vi "TagDB-Obtain.vi"(4 "error in (no error)":errorcluster, 6 "name (unnamed)":string) -> (0 "error out":errorcluster, 1 "created new?":bool, 3 "TagDB":refnum<k1>)   [LabVIEW 2017, in "TagDB.lvlib"]
uses:
  TagDB.lvlib
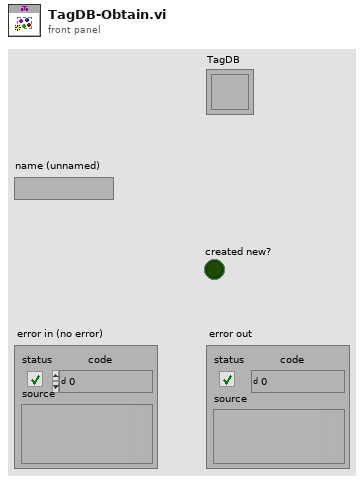
[diagram p1: front panel]
types:
  T1 = enum16{"create", "destroy", "cleanUp", "list", "get info", "force destroy"}
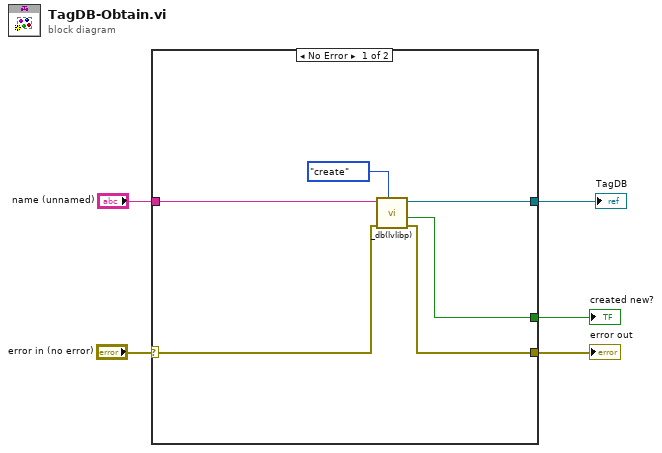
[diagram p0: block diagram]
diagram:
  n1 = case shown="No Error" "error in (no error)" {
    selector: "error in (no error)" -> [w6 w12]
    tunnel: [w10 w12] -> w2
    tunnel: [w9 _] -> w1
    tunnel: [w11 _] -> w3
    tunnel: "name (unnamed)" -> [w7 _]
    frame No Error {
      n2 = call "_db(lvlibp).vi"("command"=T1."create", "error in (no error)"=w6, "name"=w7) -> ("error out"=w10:errorcluster, "created new?"=w9:bool, "db out"=w11:refnum<k1>)  [unwired: 4 in, 2 out]
    }
    frame Error {
    }
  }
  "error out" <- w2
  "TagDB" <- w3
  "created new?" <- w1
